vi "Add Single Wheel to Steering Frame.vi"(5 "x position":dbl, 6 "frame angle (rad)":dbl, 7 "y position":dbl, 8 "error in (no error)":errorcluster, 10 "wheel":refnum<class "NI_Robotics_Wheel.lvclass">, 11 "steering frame in":refnum<class "NI_Robotics_Steering Frame.lvclass">) -> (0 "error out":errorcluster, 3 "steering frame out":refnum<class "NI_Robotics_Steering Frame.lvclass">)   [LabVIEW 2017, in "NI_Robotics_Steering Frame.lvclass"]
doc: "Adds the wheel or wheels you specify to <B>steering frame in</B>. You must manually select the polymorphic instance to use."
uses:
  <vilib>/robotics/Steering/Steering Frame/NI_Robotics_Steering Frame.lvclass
  <vilib>/robotics/Steering/Wheel/NI_Robotics_Wheel.lvclass
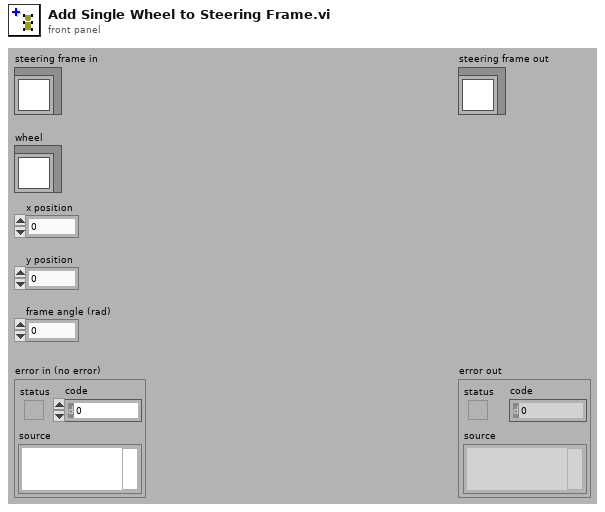
[diagram p1: front panel]
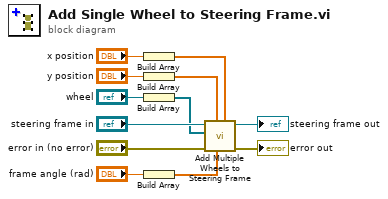
[diagram p0: block diagram]
diagram:
  n1 = Build Array("x position") -> (w4:dbl[])
  n2 = Build Array("y position") -> (w5:dbl[])
  n3 = Build Array("wheel") -> (w8:refnum<class "NI_Robotics_Wheel.lvclass">[])
  n4 = Build Array("frame angle (rad)") -> (w1:dbl[])
  n5 = call <vilib>:"Add Multiple Wheels to Steering Frame.vi"("x positions"=w4, "frame angles (rad)"=w1, "y positions"=w5, "error in (no error)"="error in (no error)", "wheels"=w8, "steering frame in"="steering frame in") -> ("error out"=→"error out":errorcluster, "steering frame out"=→"steering frame out":refnum<class "NI_Robotics_Steering Frame.lvclass">)  [unwired: 4 in]
